vi "zadanie_4.vi"() -> ()   [LabVIEW 2020]
panel:
  in  "Poziom paliwa [%]":dbl(knob) min=0.0 max=100.0 scale=0.0..100.0
  in  "Poziom maksymalny [%]":dbl min=0.0 max=100.0
  out "zbiornik":dbl(slide) scale=0.0..5.0
  out "Sygnalizacja osiagniecia\npoziomu maksymalnego":bool
  out "Sygnalizacja wlaczenia pompy":bool
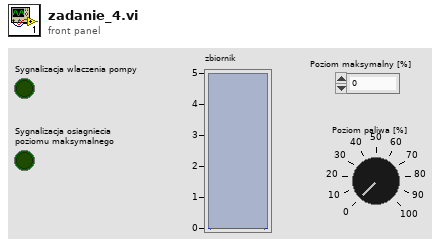
[diagram p1: front panel]
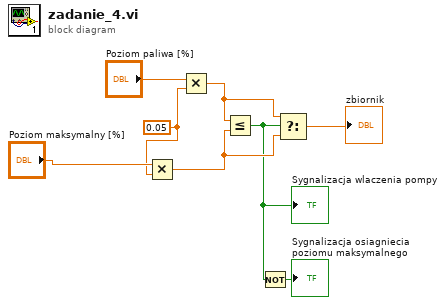
[diagram p0: block diagram]
diagram:
  w6 = 0.05
  n1 = Multiply(x="Poziom maksymalny [%]", y=w6) -> (x*y=w4:dbl)
  n2 = Multiply(x="Poziom paliwa [%]", y=w6) -> (x*y=w5:dbl)
  n3 = Less Or Equal?(x=w5, y=w4) -> (x <= y?=w3:bool)
  "Sygnalizacja wlaczenia pompy" <- w3
  n4 = Not(x=w3) -> (.not. x?=→"Sygnalizacja osiagniecia\npoziomu maksymalnego":bool)
  n5 = Select(t=w5, s=w3, f=w4) -> (s? t:f=→"zbiornik":dbl)
